vi "OnByte.vi"(8 "Uart Input":cluster{u64} {"?" format="%x"}, 11 "Error Input":errorcluster) -> (0 "Uart Output":cluster{u64} {"?" format="%x"}, 2 "On Byte Event":refnum<event-registration>, 3 "Error Output":errorcluster)   [LabVIEW 2019]
doc: "Add an <B>On Byte Received</B> event listener to the serial port."
uses:
  D:/Google Drive/INC-2020/INC352/INC352-2020/LabVIEW/examples/uart-cmdex/SubVI/dll/LabViewUart.dll
panel:
  # "Add an On_Byte event listenner"
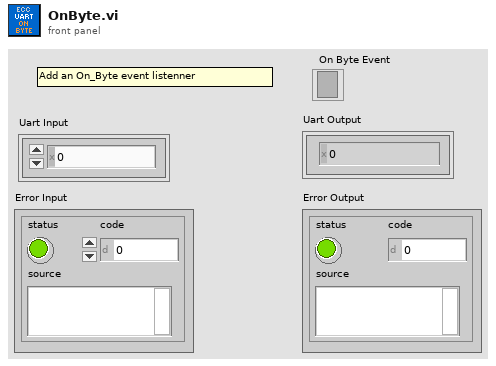
[diagram p1: front panel]
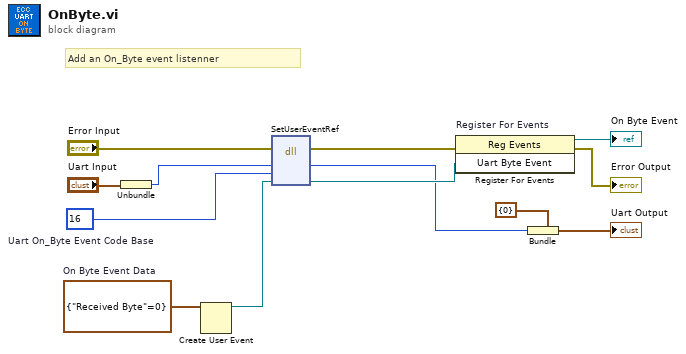
[diagram p0: block diagram]
diagram:
  w12 = u16 16  # Uart On_Byte Event Code Base
  w9 = cluster{"Received Byte":u8} {"Received Byte"=0}  # On Byte Event Data
  # "Add an On_Byte event listenner"
  n1 = Unbundle("Uart Input") -> (w1:u64)
  n2 = Create User Event(user event datatype=w9) -> (user event=w10:refnum<user-event>)  [unwired: 1 in, 1 out]
  n3 = dll-call lib="D:/Google Drive/INC-2020/INC352/INC352-2020/LabVIEW/examples/uart-cmdex/SubVI/dll/LabViewUart.dll" fn="SetUserEventRef"(error in="Error Input", "Uart Handle"=w1, "Uart On Byte Event Code Base"=w12, "Uart Byte Event"=w10) -> (error out=w7:errorcluster, "Uart Handle"=w2:u64, "Uart Byte Event"=w11:refnum<user-event>)  [unwired: 4 in, 1 out]
  n4 = register-events "Register For Events"(error in=w7, w11) -> (reference out=→"On Byte Event":refnum<event-registration>, error out=→"Error Output":errorcluster)  [unwired: 1 in]
  n5 = Bundle(cluster=cluster{u64} {0}, w2) -> (→"Uart Output":cluster{u64})
